vi "Demo_read_Write_file.vi"() -> ()   [LabVIEW 2018]
uses:
  7b35b479-6304-4ef6-8ed0-4c97cb41553a.vi
panel:
  out "Liste_mix":string[](array[string])
  in  "stop":bool
  out "Liste":string[](array[string])
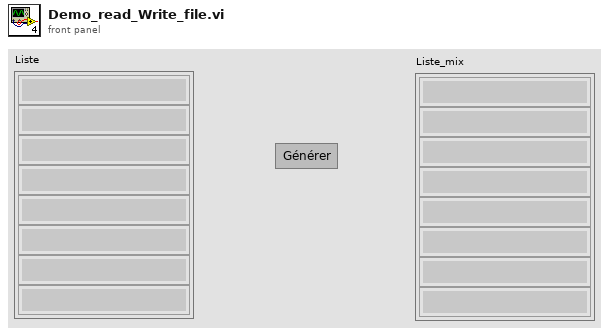
[diagram p1: front panel]
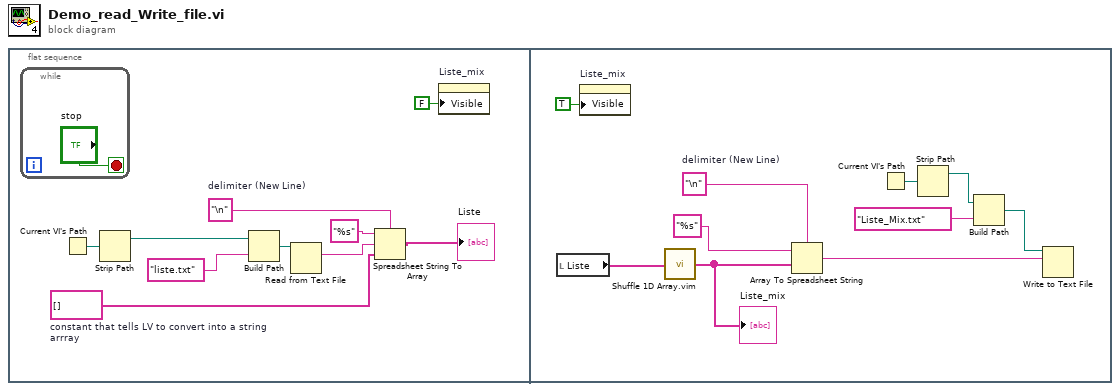
[diagram p0: block diagram]
diagram:
  n1 = flat-sequence {
    frame #0 {
      w8 = "\n"  # delimiter (New Line)
      w10 = string[] []  # constant that tells LV to convert into a string arrray
      n2 = while {
        stop <- "stop" stop-if-true
      }
      n3 = Current VI's Path() -> (path=w5:path)
      n4 = Strip Path(path=w5) -> (stripped path=w4:path)  [unwired: 1 out]
      n5 = Build Path(base path=w4, name or relative path="liste.txt") -> (appended path=w6:path)
      n6 = Read from Text File(file (use dialog)=w6) -> (text=w3:string)  [unwired: 3 in, 3 out]
      n7 = Spreadsheet String To Array(delimiter (Tab)=w8, format string="%s", spreadsheet string=w3, array type (2D Dbl)=w10) -> (array=→"Liste":string[])
      n8 = property on="Liste_mix" class="Arr (strict)"("Visible"=FALSE) -> ()  [unwired: 2 in, 2 out]
    }
    frame #1 {
      w16 = "\n"  # delimiter (New Line)
      n9 = local read "Liste"() -> (w14:string[])
      n10 = property on="Liste_mix" class="Arr (strict)"("Visible"=TRUE) -> ()  [unwired: 2 in, 2 out]
      n11 = call "Shuffle 1D Array.vim"("array"=w14) -> ("shuffled array"=w13:string[])  [unwired: 4 in]
      "Liste_mix" <- w13
      n12 = Array To Spreadsheet String(delimiter (Tab)=w16, array=w13, 3:"%s" ("format string")) -> (spreadsheet string=w17:string)
      n13 = Current VI's Path() -> (path=w20:path)
      n14 = Strip Path(path=w20) -> (stripped path=w21:path)  [unwired: 1 out]
      n15 = Build Path(base path=w21, name or relative path="Liste_Mix.txt") -> (appended path=w18:path)
      n16 = Write to Text File(file (use dialog)=w18, text=w17) -> ()  [unwired: 2 in, 3 out]
    }
  }
